vi "Get Axis Position.vi"(8 "Error In":errorcluster, 9 "Axis Enum":T1=enum."Z-axis") -> (0 "Error Out":errorcluster, 1 "Axis Enum Out":T1=enum."Z-axis", 2 "Axis Encoder Counts":i32, 3 "Axis Inches":dbl)   [LabVIEW 2013]
doc: "This sub-VI uses axis and byte select flags to communicate with an Arduino that is keeping track of up\nto four quadrature encoders. This sub-VI specifies which axis it wants to read the position of, and then\nchecks each byte of the 32-bit (4-byte) position sequentially. Finally it stores the full 32-bit position\nas an integer and outputs it."
uses:
  Controls/table_axis_enum.ctl
  <vilib>/DAQmx/write.llb/DAQmx Write (Digital 1D Bool NChan 1Samp 1Line).vi
  <vilib>/DAQmx/write.llb/DAQmx Write (Digital Bool 1Line 1Point).vi
  <vilib>/DAQmx/read.llb/DAQmx Read (Digital U8 1Chan 1Samp).vi
  <vilib>/DAQmx/miscellaneous.llb/DAQmx Fill In Error Info.vi
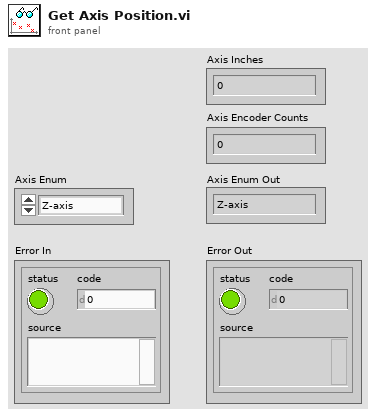
[diagram p1: front panel]
types:
  T1 = typedef "table_axis_enum.ctl" = enum16{"X-axis", "Y-axis", "Z-axis", "W-axis"}
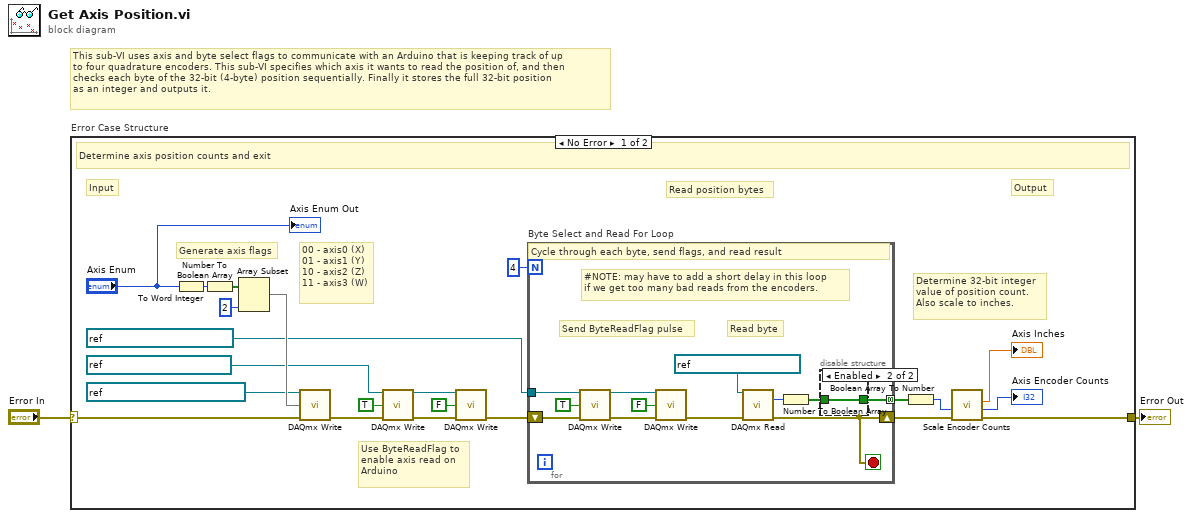
[diagram p0: block diagram]
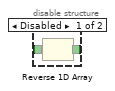
[diagram p2: hidden frame]
diagram:
  # "This sub-VI uses axis and byte select flags to communicate with an Arduino that is keeping track of up\nto four quadrature encoders. This sub-VI specifies which axis it wants to read the position of, and then\nchecks each byte of the 32-bit (4-byte) position sequentially. Finally it stores the full 32-bit position\nas an integer and outputs it."
  n1 = case "Error Case Structure" shown="No Error" "Error In" {
    selector: "Error In" -> [w12 w40]
    tunnel: [w6 w40] -> w1
    frame No Error {
      # "Input"
      # "Output"
      # "Use ByteReadFlag to\nenable axis read on\nArduino"
      # "00 - axis0 (X)\n01 - axis1 (Y)\n10 - axis2 (Z)\n11 - axis3 (W)"
      # "Generate axis flags"
      # "Determine 32-bit integer\nvalue of position count.\nAlso scale to inches."
      # "Read position bytes"
      # "Determine axis position counts and exit"
      n2 = To Word Integer(number="Axis Enum") -> (16bit integer=w19:i16)
      n3 = Number To Boolean Array(number=w19) -> (Boolean array=w20:bool[])
      n4 = Array Subset(array=w20, length=2) -> (w23:bool[])  [unwired: 1 in]
      n5 = call-poly <vilib>:"DAQmx Write.vi"("task/channels in"=refnum<k21> "SelectAxisOut_S3P00L1-2", "data"=w23, "error in"=w12) -> ("error out"=w11:errorcluster)  [unwired: 10 in, 2 out]
      n6 = call-poly <vilib>:"DAQmx Write.vi"("task/channels in"=refnum<k21> "ReadAxisFlag_S3P00L4", "data"=TRUE, "error in"=w11) -> ("task out"=w9:refnum<k21>, "error out"=w10:errorcluster)  [unwired: 10 in, 1 out]
      n7 = call-poly <vilib>:"DAQmx Write.vi"("task/channels in"=w9, "data"=FALSE, "error in"=w10) -> ("error out"=w16:errorcluster)  [unwired: 10 in, 2 out]
      n8 = for "Byte Select and Read For Loop" {
        N: 4 -> [_]
        shift-right: [w33] -> w7
        shift-left: w16 -> [w29]
        tunnel: [w25] -> w8 mode=concatenating
        tunnel: refnum<k21> "ByteReadFlag_S3P00L3" ("task/channels in") -> [w28]
        stop <- w33 stop-if-true
        # "#NOTE: may have to add a short delay in this loop\nif we get too many bad reads from the encoders."
        # "Read byte"
        # "Send ByteReadFlag pulse"
        # "Cycle through each byte, send flags, and read result"
        n9 = call-poly <vilib>:"DAQmx Write.vi"("task/channels in"=w28, "data"=TRUE, "error in"=w29) -> ("task out"=w35:refnum<k21>, "error out"=w27:errorcluster)  [unwired: 10 in, 1 out]
        n10 = call-poly <vilib>:"DAQmx Write.vi"("task/channels in"=w35, "data"=FALSE, "error in"=w27) -> ("error out"=w34:errorcluster)  [unwired: 10 in, 2 out]
        n11 = call-poly <vilib>:"DAQmx Read.vi"("task/channels in"=refnum<k21> "EncodePosIn_S3P1", "error in"=w34) -> ("data"=w32:u8, "error out"=w33:errorcluster)  [unwired: 11 in, 1 out]
        n12 = Number To Boolean Array(number=w32) -> (Boolean array=w26:bool[])
        n13 = disable-structure shown="Enabled" {
          disable-tunnel: w26 -> [w38 w39]
          disable-tunnel: [w37 w39] -> w25
          frame Disabled {
            n14 = Reverse 1D Array(array=w38) -> (reversed array=w37:bool[])
          }
          frame Enabled {
          }
        }
      }
      n15 = Boolean Array To Number(Boolean array=w8) -> (number=w5:i32)
      n16 = call "Scale Encoder Counts.vi"("Error In"=w7, "Axis Encoder Counts"=w5) -> ("Error Out"=w6:errorcluster, "Axis Encoder Counts out"=→"Axis Encoder Counts":i32, "Axis Inches"=→"Axis Inches":dbl)  [unwired: 7 in]
      "Axis Enum Out" <- "Axis Enum"
    }
    frame Error {
      # "Pass through and exit"
    }
  }
  "Error Out" <- w1
